vi "Replace Item in Peek Stack.vi"(8 "error in (no error)":errorcluster, 11 "Data Cluster in":T1) -> (0 "error out":errorcluster, 2 "Active VI Previous State":refnum<class "Standard VI Type.lvclass">, 3 "Data Cluster out":T1)   [LabVIEW 2020, in "Peek Window.lvlib"]
uses:
  Peek Window.lvlib
  MHL Data Cluster.ctl
  VI Types/Standard VI Type/Standard VI Type.lvclass
  Open Diagram Argument--cluster.ctl
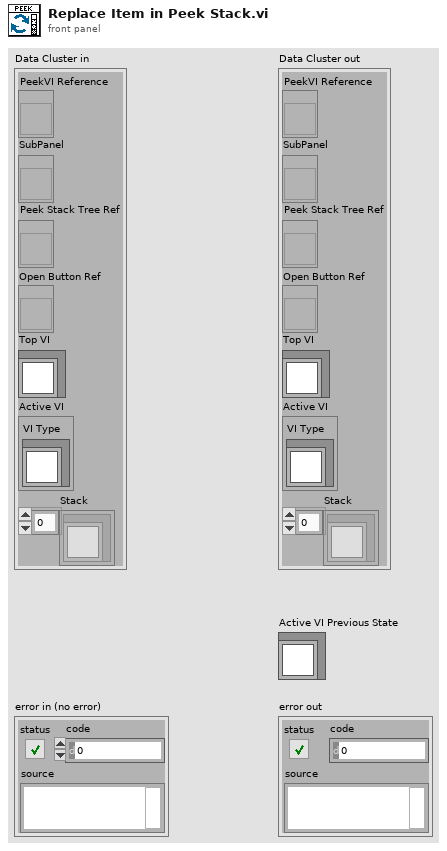
[diagram p1: front panel]
types:
  T1 = typedef "Peek Window.lvlib/MHL Data Cluster.ctl" = cluster{"PeekVI Reference":refnum<vi>, "SubPanel":refnum<vi>, "Peek Stack Tree Ref":refnum<vi>, "Open Button Ref":refnum<vi>, "Top VI":refnum<class "Standard VI Type.lvclass">, "Active VI":T2, "Stack":refnum<class "Standard VI Type.lvclass">[]}
  T2 = typedef "Peek Window.lvlib/Open Diagram Argument--cluster.ctl" = cluster{"VI Type":refnum<class "Standard VI Type.lvclass">}
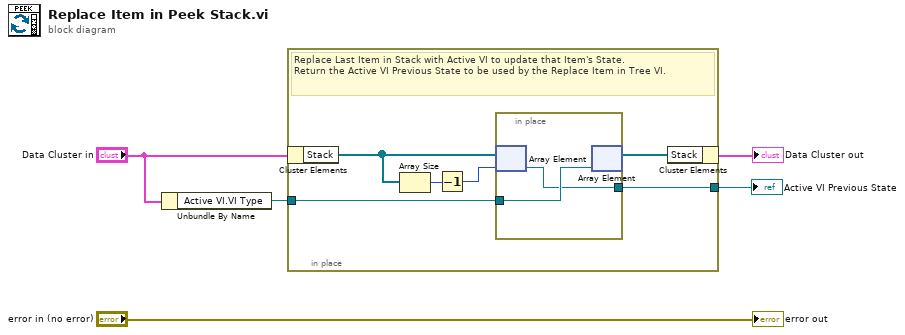
[diagram p0: block diagram]
diagram:
  n1 = Unbundle By Name("Data Cluster in") -> ("Active VI.VI Type"=w1:refnum<class "Standard VI Type.lvclass">)
  n2 = in-place {
    in-place-border: w1 -> [w8]
    in-place-border: [w6] -> w3
    # "Replace Last Item in Stack with Active VI to update that Item's State.\nReturn the Active VI Previous State to be used by the Replace Item in Tree VI."
    n3 = in-place-cluster #1("Data Cluster in") -> ("Stack"=w11:refnum<class "Standard VI Type.lvclass">[])
    n4 = Array Size(array=w11) -> (size(s)=w10:i32)
    n5 = Decrement(x=w10) -> (x-1=w9:i32)
    n6 = in-place {
      in-place-border: w8 -> [w13]
      in-place-border: [w12] -> w6
      n7 = in-place-array #2(w11, w9) -> (w12:refnum<class "Standard VI Type.lvclass">)
      n8 = in-place-array #2(w13) -> (w7:refnum<class "Standard VI Type.lvclass">[])  [unwired: 1 out]
    }
    n9 = in-place-cluster #1("Stack"=w7) -> (→"Data Cluster out":T1)
  }
  "Active VI Previous State" <- w3
  "error out" <- "error in (no error)"
